vi "Waveform Data Convert.vi"(8 "error in (no error)":errorcluster, 10 "Waveform Data (Empty)":string, 11 "VISA resource name":refnum<visa-resource-name>) -> (0 "error out":errorcluster, 1 "Data Byte Number":i32, 2 "Output":dbl[](array[numeric]), 3 "VISA resource name out":refnum<visa-resource-name>)   [LabVIEW 2021, in "Yokogawa WT1800 Series.lvlib"]
doc: "Transforms acquisition waveform datas into voltage array values for the waveform graph."
uses:
  <instrlib>/Yokogawa WT1800 Series/Yokogawa WT1800 Series.lvlib
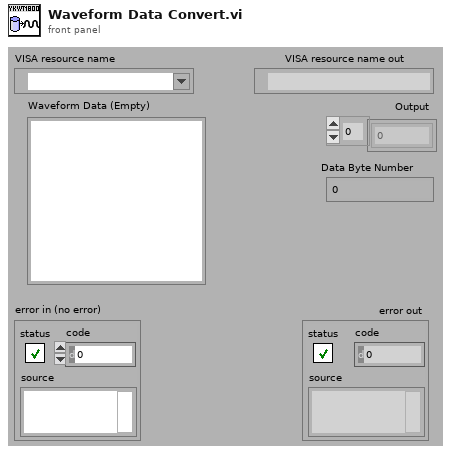
[diagram p1: front panel]
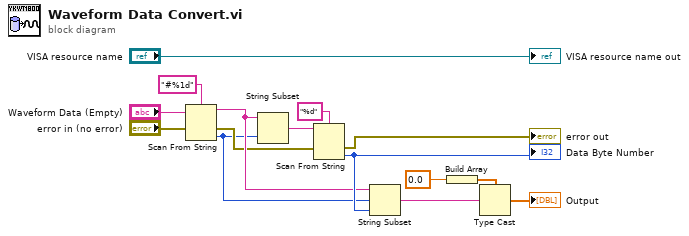
[diagram p0: block diagram]
diagram:
  n1 = Scan From String ("文字列からスキャン")(format string="#%1d", input string="Waveform Data (Empty)", error in="error in (no error)") -> (remaining string=w9:string, error out=w5:errorcluster, output 1=w1:i32)  [unwired: 2 in, 1 out]
  n2 = String Subset ("部分文字列")(string=w9, length (rest)=w1) -> (substring=w8:string)  [unwired: 1 in]
  n3 = Scan From String ("文字列からスキャン")(format string="%d", input string=w8, error in=w5) -> (error out=→"error out":errorcluster, output 1=w12:i32)  [unwired: 2 in, 2 out]
  "Data Byte Number" <- w12
  n4 = String Subset ("部分文字列")(string=w9, offset (0)=w1, length (rest)=w12) -> (substring=w2:string)
  n5 = Build Array ("配列連結追加")(sgl 0.0) -> (w4:sgl[])
  n6 = Type Cast ("タイプキャスト")(type=w4, x=w2) -> (*(type *) &x=→"Output":sgl[])
  "VISA resource name out" <- "VISA resource name"
